vi "Update IP.vi"(8 "error in":errorcluster, 11 "Message string":string) -> (0 "error out":errorcluster)   [LabVIEW 2014]
uses:
  Message Queue/Message Queue.lvlib
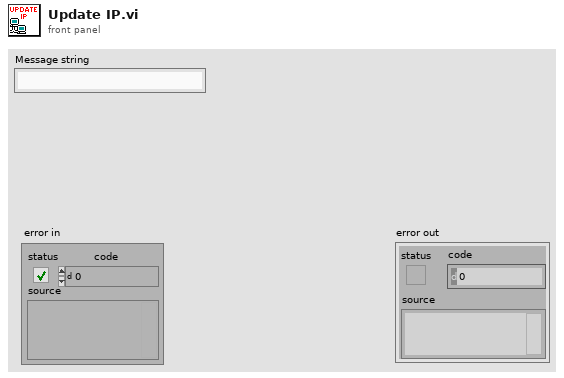
[diagram p1: front panel]
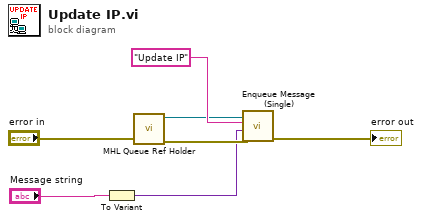
[diagram p0: block diagram]
diagram:
  n1 = To Variant(anything="Message string") -> (Variant=w1:variant)
  n2 = call "MHL Queue Ref Holder.vi"("error in"="error in") -> ("error out"=w3:errorcluster, "Input Message Queue"=w4:refnum<queue>)  [unwired: 9 in]
  n3 = call "Enqueue Message (Single).vi"("error in (no error)"=w3, "Message Data"=w1, "Message"="Update IP", "Message Queue"=w4) -> ("error out"=→"error out":errorcluster)  [unwired: 6 in, 1 out]
